vi "BRig_FPGA_v3,93.vi"() -> ()   [LabVIEW 2014]
uses:
  <vilib>/rvi/Emulation/niFpgaGetClockAttributes.vi
  <vilib>/rvi/Emulation/niFpgaSctlEmulationGetInTimedLoop.vi
  <vilib>/rvi/Emulation/niFpgaEmulationReportErrorSimple.vi
  <vilib>/rvi/eio/common/nirviEmuTemplateMethod_errors.vi
  <vilib>/rvi/Emulation/niFpgaCriticalErrorInLSC.vi
  <vilib>/eio/EIONode/EIONode.xnode
panel:
  out "fpga_solenoid_R":bool
  out "fpga_solenoid_L":bool
  out "fpga_laser2":bool
  out "fpga_laser1":bool
  in  "L2Led_ON":bool
  in  "L1Led_ON":bool
  in  "Rising(F)_or_Falling(T)":bool
  in  "Solenoid_trig_R":bool
  in  "Solenoid_trig_L":bool
  in  "Solenoid_nTotal_R":u32=100
  in  "Solenoid_nTotal_L":u32=100
  in  "L2Led_Baseline":bool
  in  "L1Led_Baseline":bool
  in  "CueLed_Baseline":bool
  in  "I_allReward":bool
  in  "AnaOut_1":u16
  in  "CueLed_Event":bool
  in  "CueLed_nValley":u32=100
  in  "CueLed_nPeak":u32=100
  in  "LC_Event_l2":bool
  in  "LC_Laser_l2":bool
  in  "LC_nShutter_l2":u32=100
  in  "LC_nValley_l2":u32=100
  in  "LC_nPeak_l2":u32=100
  in  "LR_wrong_nDelay_l2":u32
  in  "LR_reward_nDelay_l2":u32
  in  "LR_wrong_nTotal_l2":u32=100
  in  "LR_reward_nTotal_l2":u32=100
  in  "LR_wrong_laser_l2":bool
  in  "LR_wrong_Event_l2":bool
  in  "LR_reward_Laser_l2":bool
  in  "LR_reward_Event_l2":bool
  out "AnaIn_1":u16
  out "AnaIn_0":u16
  out "timeTrial_count":u32
  in  "timeTrial_trig":bool
  in  "k1__counter_per_ms":u16=100 min=100 max=40000 step=1
  in  "LC_nShutter_l1":u32=100
  in  "AnaOut_0":u16
  in  "LC_nValley_l1":u32=100
  in  "LC_nPeak_l1":u32=100
  in  "LC_Event_l1":bool
  in  "LR_wrong_nTotal_l1":u32=100
  in  "LR_wrong_nDelay_l1":u32
  in  "LR_reward_nTotal_l1":u32=100
  in  "LR_reward_nDelay_l1":u32
  in  "LR_reward_Event_l1":bool
  in  "LR_wrong_Event_l1":bool
  out "SelectWrong":bool
  out "SelectReward":bool
  in  "LR_wrong_Laser_l1":bool
  in  "LR_reward_Laser_l1":bool
  in  "Left(F)_or_Right(T)":bool
  in  "ignoreWrong":bool
  in  "SelectionState":bool
  in  "LC_Laser_l1":bool
  in  "FPGA_Stop":bool
  in  "audioTrigger_L":bool
  in  "audioTrigger_R":bool
  in  "audioFreq_L_kHz":u8=14 min=1 max=14 step=1
  in  "audioAmp_L":u16=1 min=1 max=32767 step=1
  in  "audioFreq_R_kHz":u8=14 min=1 max=14 step=1
  in  "audioAmp_R":u16=1 min=1 max=32767 step=1
  in  "A3_SL":bool
  in  "A1_SR":bool
  in  "Counts_Reset":bool
  out "A4_LickR":u32
  out "A2_LickL":u32
  in  "A6_Act":bool
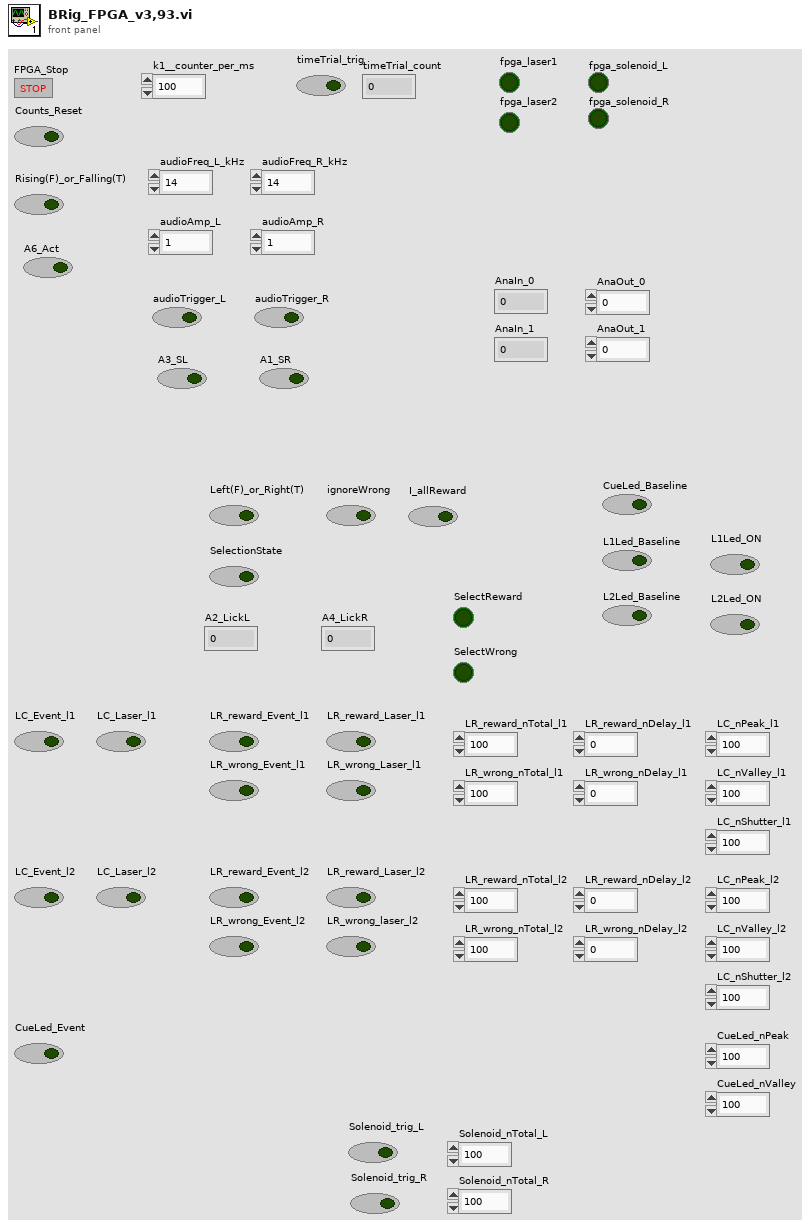
[diagram p1: front panel]
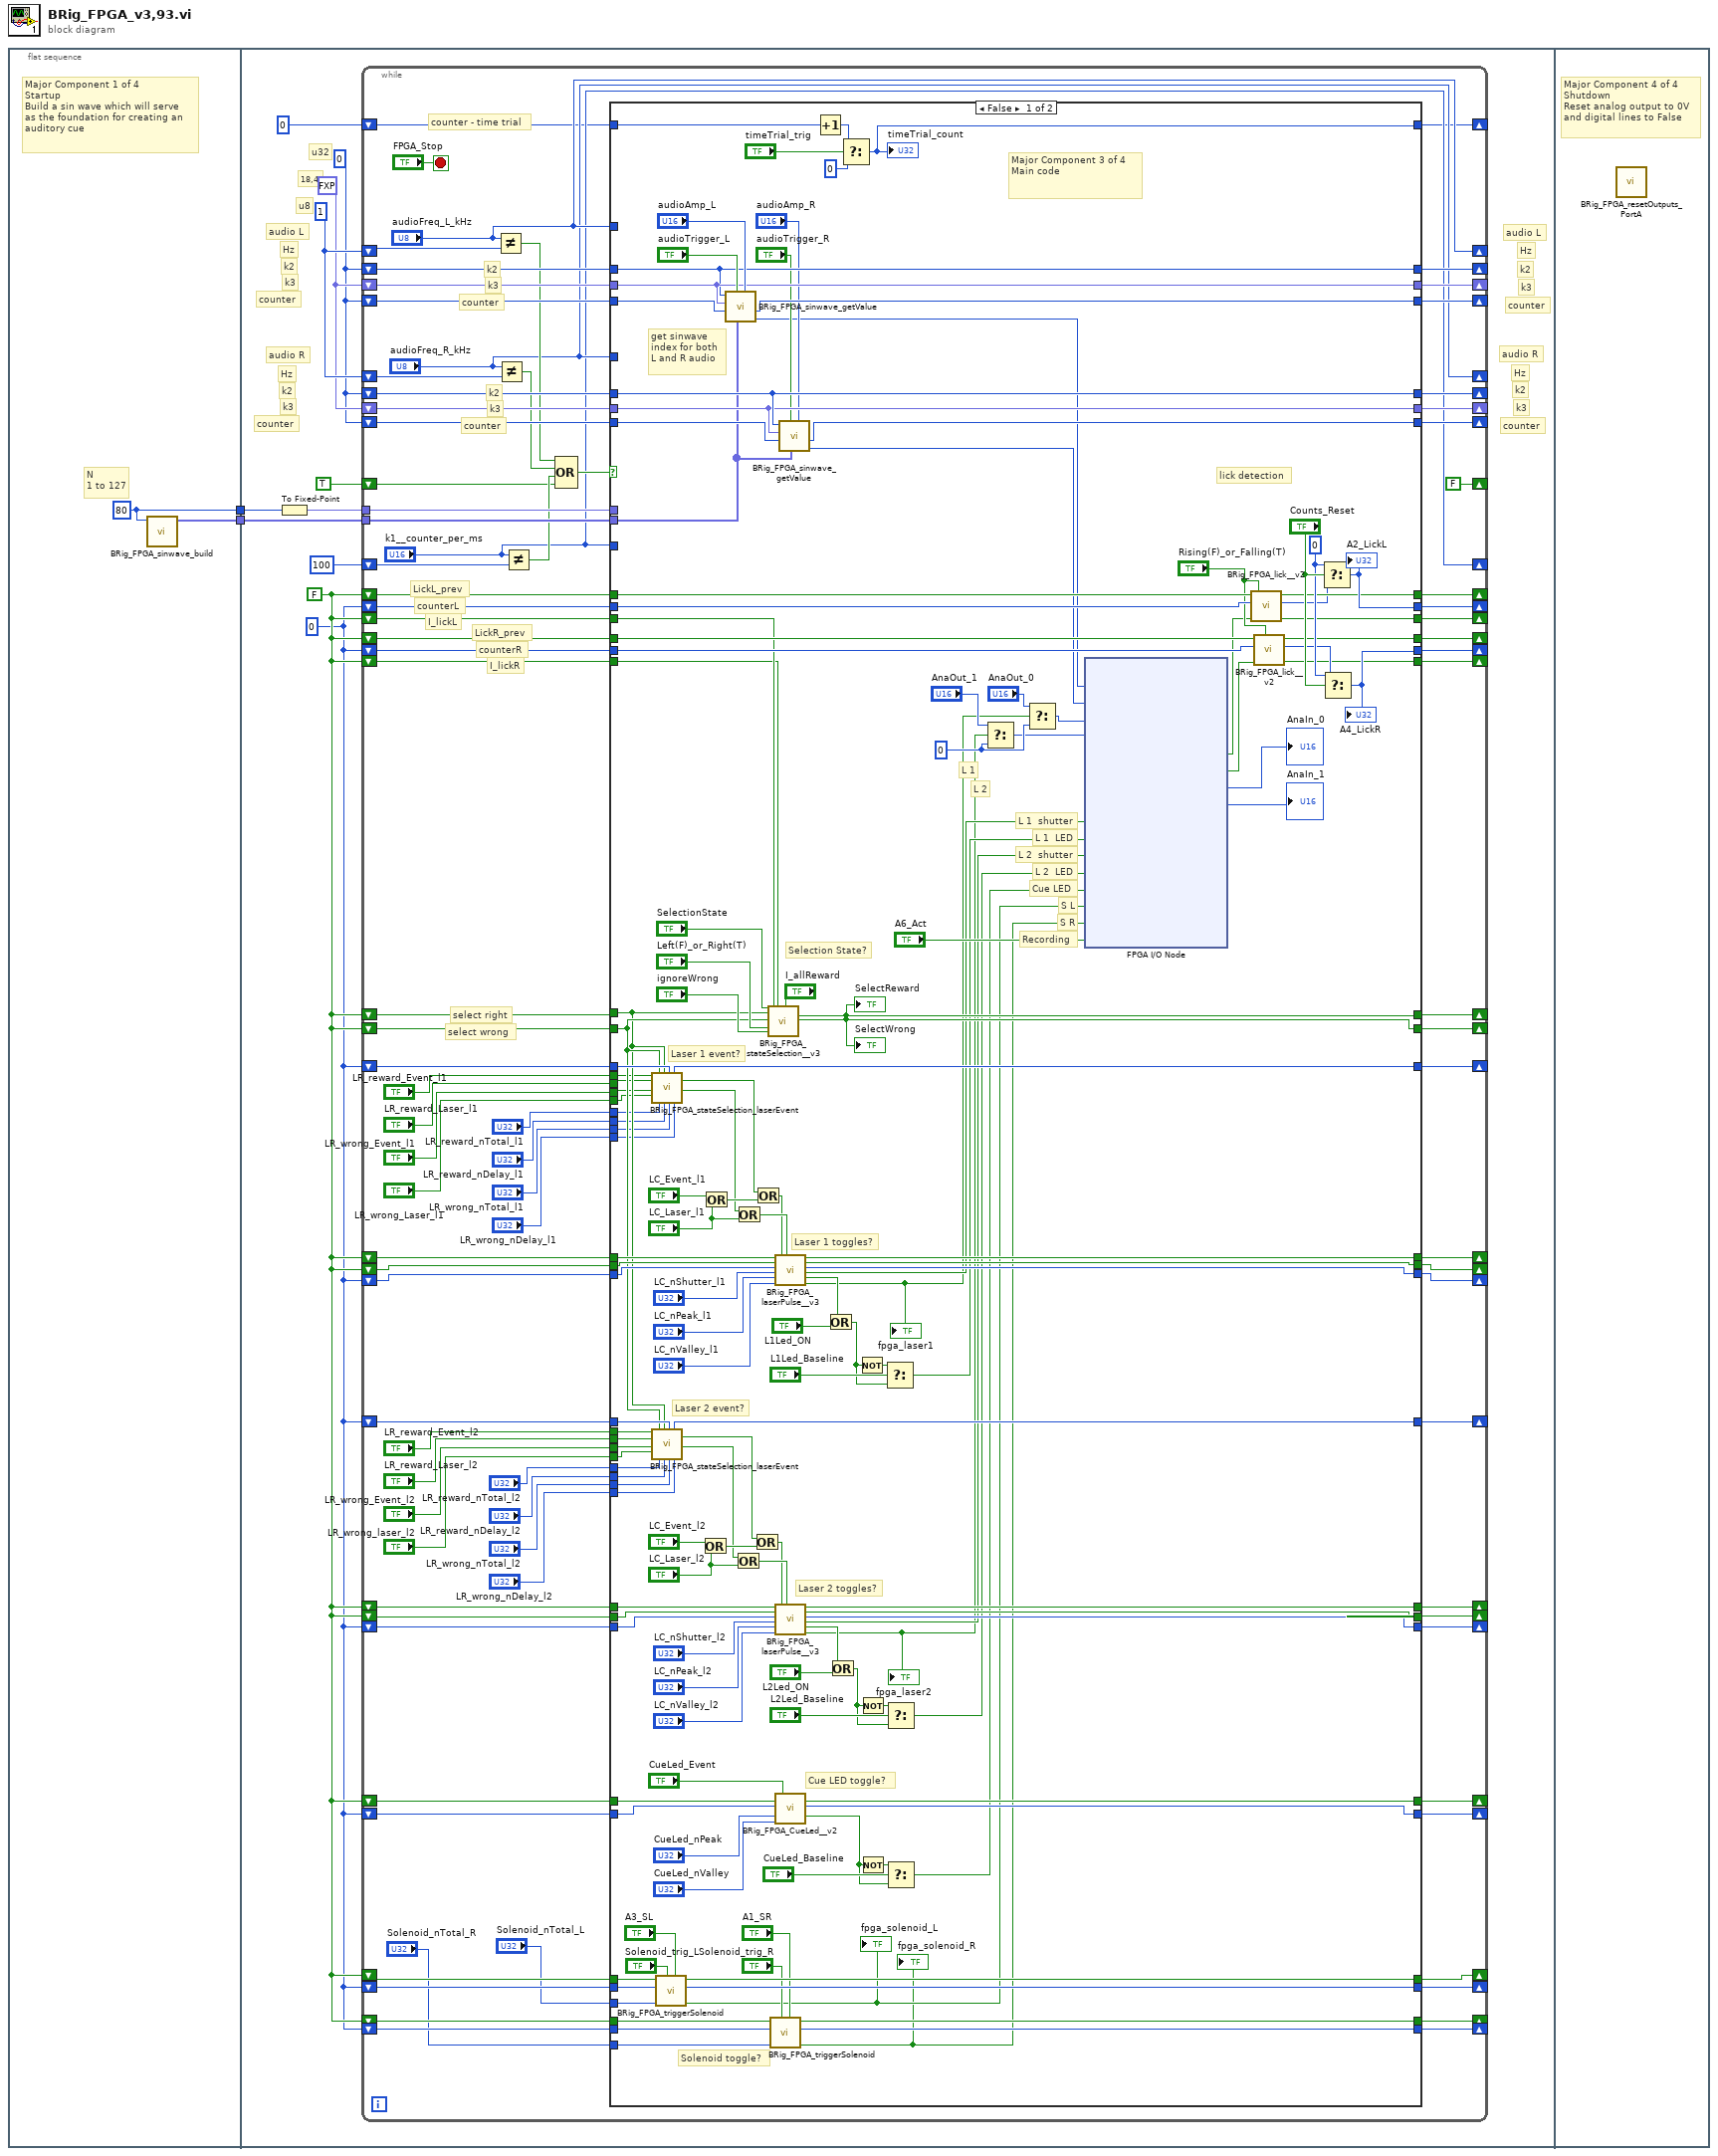
[diagram p0: block diagram]
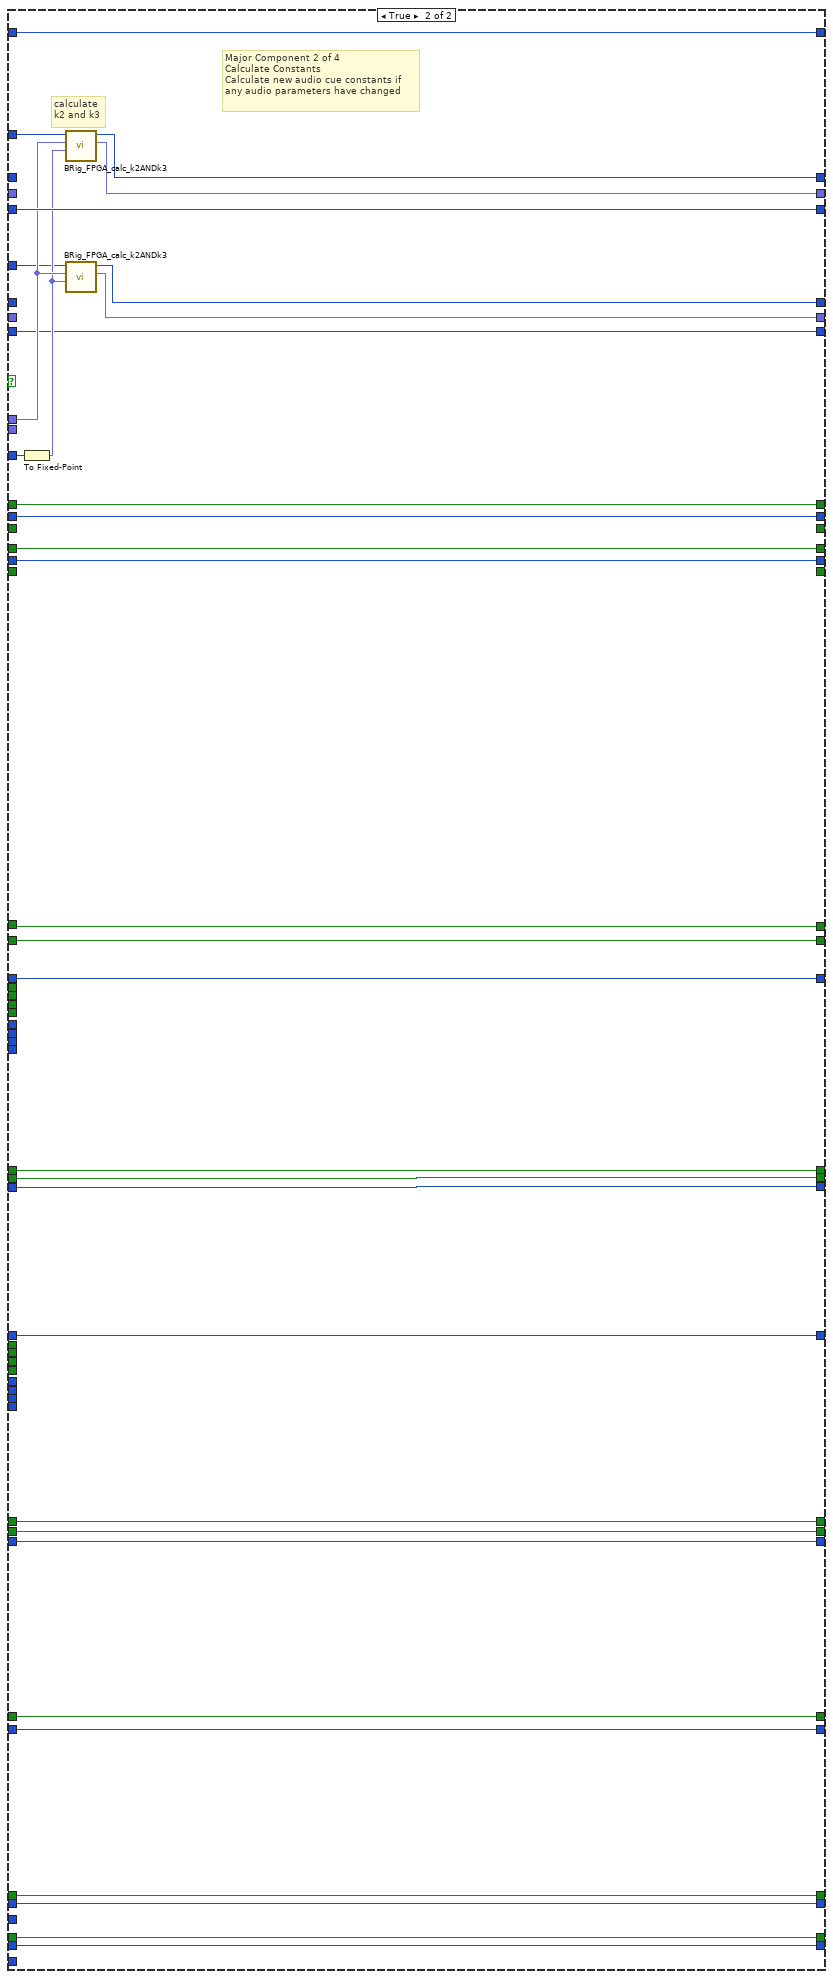
[diagram p2: hidden frame]
diagram:
  n1 = flat-sequence {
    tunnel: [w4] -> w2
    tunnel: [w3] -> w1
    tunnel: w2 -> [w15]
    tunnel: w1 -> [w14]
    frame #0 {
      w3 = 80 ("dimension size")
      # "Major Component 1 of 4\nStartup\nBuild a sin wave which will serve\nas the foundation for creating an\nauditory cue"
      # "N\n1 to 127"
      n2 = call "BRig_FPGA_sinwave_build.vi"("input_Npts"=w3) -> ("output_array_sin"=w4:fxp<+/-,16,2>[])  [unwired: 10 in]
    }
    frame #1 {
      w5 = u32 0
      w6 = FALSE
      w10 = u32 0
      w11 = fxp<+,18,4> 0.0
      w12 = u8 1
      # "counter"
      # "k3"
      # "k2"
      # "counter"
      # "k3"
      # "k2"
      # "counter"
      # "counter"
      # "u32"
      # "k3"
      # "k2"
      # "k3"
      # "18,4"
      # "u8"
      # "Hz"
      # "Hz"
      # "audio R"
      # "audio L"
      # "Hz"
      # "k2"
      # "Hz"
      # "audio R"
      # "audio L"
      n3 = To Fixed-Point(number=w14) -> (fixed-point=w13:fxp<+,7,7>)  [unwired: 1 in]
      n4 = while {
        shift-right: ["audioFreq_L_kHz"] -> _
        shift-left: w12 -> [w106]
        shift-right: [w100] -> _
        shift-left: w10 -> [w104]
        shift-right: ["audioFreq_R_kHz"] -> _
        shift-left: w12 -> [w96]
        tunnel: w15 -> [w103]
        tunnel: w13 -> [w102]
        shift-right: [w99] -> _
        shift-left: w11 -> [w101]
        shift-right: [w97] -> _
        shift-left: w10 -> [w98]
        shift-right: [w94] -> _
        shift-left: w10 -> [w95]
        shift-right: [w92] -> _
        shift-left: w11 -> [w93]
        shift-right: [w90] -> _
        shift-left: w10 -> [w91]
        shift-right: ["k1__counter_per_ms"] -> _
        shift-left: u16 100 ("y") -> [w89]
        shift-right: [FALSE] -> _
        shift-left: TRUE -> [w84]
        shift-right: [w77] -> _
        shift-left: w6 -> [w79]
        shift-right: [w76] -> _
        shift-left: w6 -> [w78]
        shift-right: [w74] -> _
        shift-left: w5 -> [w75]
        shift-right: [w72] -> _
        shift-left: w5 -> [w73]
        shift-right: [w69] -> _
        shift-left: w6 -> [w71]
        shift-right: [w68] -> _
        shift-left: w6 -> [w70]
        shift-right: [w66] -> _
        shift-left: w6 -> [w67]
        shift-right: [w64] -> _
        shift-left: w6 -> [w65]
        shift-right: [w62] -> _
        shift-left: u32 0 -> [w63]
        shift-right: [w60] -> _
        shift-left: w5 -> [w61]
        shift-right: [w59] -> _
        shift-left: w6 -> [w56]
        shift-right: [w58] -> _
        shift-left: w6 -> [w55]
        shift-right: [w57] -> _
        shift-left: w5 -> [w54]
        shift-right: [w52] -> _
        shift-left: w5 -> [w53]
        shift-right: [w51] -> _
        shift-left: w6 -> [w48]
        shift-right: [w50] -> _
        shift-left: w6 -> [w47]
        shift-right: [w49] -> _
        shift-left: w5 -> [w46]
        shift-right: [w45] -> _
        shift-left: w6 -> [w43]
        shift-right: [w44] -> _
        shift-left: w5 -> [w42]
        shift-right: [w24] -> _
        shift-left: w5 -> [w25]
        shift-right: [w21] -> _
        shift-left: w6 -> [w23]
        shift-right: [w18] -> _
        shift-left: w6 -> [w20]
        shift-right: [w17] -> _
        shift-left: w5 -> [w19]
        stop <- "FPGA_Stop" stop-if-true
        # "counter"
        # "k3"
        # "k2"
        # "counter"
        # "k3"
        # "k2"
        # "counter - time trial"
        # "I_lickR"
        # "counterR"
        # "LickR_prev"
        # "I_lickL"
        # "counterL"
        # "LickL_prev"
        # "select wrong"
        # "select right"
        n5 = Not Equal?(x="audioFreq_L_kHz", y=w106) -> (x != y?=w88:bool)
        n6 = Not Equal?(x="audioFreq_R_kHz", y=w96) -> (x != y?=w87:bool)
        n7 = Not Equal?(x="k1__counter_per_ms", y=w89) -> (x != y?=w85:bool)
        n8 = Compound Arithmetic op=OR(w88, w87, w85, w84) -> (w86:bool)
        n9 = case shown="False" w86 {
          tunnel: w104 -> [w241 _]
          tunnel: "audioFreq_L_kHz" -> [_ w287]
          tunnel: w103 -> [w234 _]
          tunnel: w102 -> [_ w283]
          tunnel: "k1__counter_per_ms" -> [_ w288]
          tunnel: w101 -> [w242 _]
          tunnel: [w241 w286] -> w100
          tunnel: [w242 w285] -> w99
          tunnel: w98 -> [w246 w284]
          tunnel: [w243 w284] -> w97
          tunnel: w95 -> [w238 _]
          tunnel: [w238 w279] -> w94
          tunnel: w93 -> [w237 _]
          tunnel: [w237 w280] -> w92
          tunnel: w91 -> [w240 w278]
          tunnel: "audioFreq_R_kHz" -> [_ w281]
          tunnel: [w239 w278] -> w90
          tunnel: w79 -> [w229 w277]
          tunnel: w78 -> [w228 w276]
          tunnel: [w233 w277] -> w77
          tunnel: [w226 w276] -> w76
          tunnel: w75 -> [w230 w275]
          tunnel: [w256 w275] -> w74
          tunnel: w73 -> [w227 w274]
          tunnel: [w253 w274] -> w72
          tunnel: w71 -> [w184 w273]
          tunnel: w70 -> [w185 w272]
          tunnel: [w204 w273] -> w69
          tunnel: [w249 w272] -> w68
          tunnel: [w219 w269] -> w59
          tunnel: [w220 w268] -> w58
          tunnel: [w221 w267] -> w57
          tunnel: w67 -> [w223 _]
          tunnel: [w232 _] -> w66
          tunnel: w65 -> [w222 _]
          tunnel: [w224 _] -> w64
          tunnel: w63 -> [w211 w271]
          tunnel: [w208 w271] -> w62
          tunnel: w61 -> [w203 w270]
          tunnel: [w202 w270] -> w60
          tunnel: w56 -> [w201 w269]
          tunnel: w55 -> [w200 w268]
          tunnel: w54 -> [w199 w267]
          tunnel: w53 -> [w187 w266]
          tunnel: [w186 w266] -> w52
          tunnel: [w182 w265] -> w51
          tunnel: [w181 w264] -> w50
          tunnel: [w180 w263] -> w49
          tunnel: w48 -> [w179 w265]
          tunnel: w47 -> [w178 w264]
          tunnel: w46 -> [w177 w263]
          tunnel: [w174 w262] -> w45
          tunnel: [w173 w261] -> w44
          tunnel: w43 -> [w172 w262]
          tunnel: w42 -> [w171 w261]
          tunnel: "LR_reward_Event_l1" -> [w157 _]
          tunnel: "LR_reward_Laser_l1" -> [w156 _]
          tunnel: "LR_wrong_Event_l1" -> [w155 _]
          tunnel: "LR_wrong_Laser_l1" -> [w154 _]
          tunnel: "LR_reward_nTotal_l1" -> [w153 _]
          tunnel: "LR_reward_nDelay_l1" -> [w152 _]
          tunnel: "LR_wrong_nTotal_l1" -> [w151 _]
          tunnel: "LR_wrong_nDelay_l1" -> [w150 _]
          tunnel: "LR_reward_Event_l2" -> [w149 _]
          tunnel: "LR_reward_Laser_l2" -> [w148 _]
          tunnel: "LR_wrong_Event_l2" -> [w147 _]
          tunnel: "LR_wrong_laser_l2" -> [w146 _]
          tunnel: "LR_reward_nTotal_l2" -> [w145 _]
          tunnel: "LR_reward_nDelay_l2" -> [w144 _]
          tunnel: "LR_wrong_nTotal_l2" -> [w143 _]
          tunnel: "LR_wrong_nDelay_l2" -> [w142 _]
          tunnel: w25 -> [w141 w260]
          tunnel: [w136 w260] -> w24
          tunnel: w23 -> [w140 w259]
          tunnel: "Solenoid_nTotal_L" -> [w139 _]
          tunnel: [w135 w259] -> w21
          tunnel: w20 -> [w132 w258]
          tunnel: w19 -> [w131 w257]
          tunnel: [w130 w258] -> w18
          tunnel: [w129 w257] -> w17
          tunnel: "Solenoid_nTotal_R" -> [w128 _]
          frame False {
            w168 = u16 0 ("f")
            w254 = u32 0 ("t")
            # "Cue LED"
            # "L 2  shutter"
            # "L 2  LED"
            # "L 1  shutter"
            # "L 1  LED"
            # "Recording"
            # "S L"
            # "S R"
            # "L 2"
            # "L 1"
            # "Solenoid toggle?"
            # "Cue LED toggle?"
            # "Laser 2 toggles?"
            # "Laser 2 event?"
            # "Laser 1 toggles?"
            # "Selection State?"
            # "Laser 1 event?"
            # "Major Component 3 of 4\nMain code"
            # "get sinwave\nindex for both\nL and R audio"
            # "lick detection"
            n10 = call "BRig_FPGA_stateSelection_laserEvent.vi"("I_LR_reward"=w157, "I_LR_reward_laser"=w156, "I_LR_wrong"=w155, "I_LR_wrong_laser"=w154, "I_selectWrong"=w185, "laser_reward_nTotal"=w153, "I_selectReward"=w184, "laser_reward_nDelay"=w152, "counter"=w203, "laser_wrong_nTotal"=w151, "laser_wrong_nDelay"=w150) -> ("output_counter"=w202:u32, "output_I_laserEvent"=w198:bool, "output_I_laserOn"=w197:bool)  [unwired: 6 in]
            n11 = call "BRig_FPGA_stateSelection_laserEvent.vi"("I_LR_reward"=w149, "I_LR_reward_laser"=w148, "I_LR_wrong"=w147, "I_LR_wrong_laser"=w146, "I_selectWrong"=w185, "laser_reward_nTotal"=w145, "I_selectReward"=w184, "laser_reward_nDelay"=w144, "counter"=w187, "laser_wrong_nTotal"=w143, "laser_wrong_nDelay"=w142) -> ("output_counter"=w186:u32, "output_I_laserEvent"=w183:bool, "output_I_laserOn"=w188:bool)  [unwired: 6 in]
            n12 = call "BRig_FPGA_triggerSolenoid.vi"("input_Solenoid_MTrig"="A3_SL", "input_Solenoid_trig"="Solenoid_trig_L", "input_threshold"=w139, "input_counter"=w141, "input_trig"=w140) -> ("output_Solenoid_OnOff"=w108:bool, "output_counter"=w136:u32, "output_trig"=w135:bool)  [unwired: 4 in]
            "fpga_solenoid_L" <- w108
            n13 = Or(x="LC_Event_l2", y="LC_Laser_l2") -> (x .or. y?=w192:bool)
            n14 = Or(x="LC_Event_l1", y="LC_Laser_l1") -> (x .or. y?=w215:bool)
            n15 = call "BRig_FPGA_sinwave_getValue.vi"("audioAmp"="audioAmp_L", "sinwave"=w234, "audioTrigger"="audioTrigger_L", "counter"=w246, "k3"=w242, "k2"=w241) -> ("output_audioValue"=w206:i16, "output_counter"=w243:u32)  [unwired: 4 in]
            n16 = Or(x=w188, y="LC_Laser_l2") -> (x .or. y?=w190:bool)
            n17 = Or(x=w197, y="LC_Laser_l1") -> (x .or. y?=w213:bool)
            n18 = Or(x=w183, y=w192) -> (x .or. y?=w189:bool)
            n19 = Or(x=w198, y=w215) -> (x .or. y?=w212:bool)
            n20 = call "BRig_FPGA_stateSelection__v3.vi"("I_selectionState"="SelectionState", "I_selectRight"=w184, "I_selectWrong"=w185, "I_Left(F)_or_Right(T)"="Left(F)_or_Right(T)", "I_ignoreWrong"="ignoreWrong", "I_lickL"=w223, "I_lickR"=w222, "I_allReward"="I_allReward") -> ("output__I_selectRight"=w204:bool, "output__I_selectWrong"=w249:bool)  [unwired: 18 in]
            "SelectWrong" <- w249
            "SelectReward" <- w204
            n21 = call "BRig_FPGA_triggerSolenoid.vi"("input_Solenoid_MTrig"="A1_SR", "input_Solenoid_trig"="Solenoid_trig_R", "input_threshold"=w128, "input_counter"=w131, "input_trig"=w132) -> ("output_Solenoid_OnOff"=w107:bool, "output_counter"=w129:u32, "output_trig"=w130:bool)  [unwired: 4 in]
            "fpga_solenoid_R" <- w107
            n22 = call "BRig_FPGA_laserPulse__v3.vi"("I_shutter"=w201, "I_peak"=w200, "count"=w199, "laser_Nshutter"="LC_nShutter_l1", "laser_Npeak"="LC_nPeak_l1", "laser_Nvalley"="LC_nValley_l1", "I_laserEvent"=w212, "I_laser"=w213) -> ("output_I_shutter"=w219:bool, "output_I_peak"=w220:bool, "output_count"=w221:u32, "output_shutter"=w115:bool, "output_led"=w125:bool, "output_laser"=w110:bool)  [unwired: 6 in]
            "fpga_laser1" <- w110
            n23 = call "BRig_FPGA_laserPulse__v3.vi"("I_shutter"=w179, "I_peak"=w178, "count"=w177, "laser_Nshutter"="LC_nShutter_l2", "laser_Npeak"="LC_nPeak_l2", "laser_Nvalley"="LC_nValley_l2", "I_laserEvent"=w189, "I_laser"=w190) -> ("output_I_shutter"=w182:bool, "output_I_peak"=w181:bool, "output_count"=w180:u32, "output_shutter"=w113:bool, "output_led"=w122:bool, "output_laser"=w109:bool)  [unwired: 6 in]
            "fpga_laser2" <- w109
            n24 = call "BRig_FPGA_CueLed__v2.vi"("I_peak"=w172, "count"=w171, "laser_Npeak"="CueLed_nPeak", "laser_Nvalley"="CueLed_nValley", "I_CueLed_Event"="CueLed_Event") -> ("output_I_peak"=w174:bool, "output_count"=w173:u32, "output_led"=w162:bool)  [unwired: 12 in]
            n25 = call "BRig_FPGA_sinwave_getValue.vi"("audioAmp"="audioAmp_R", "sinwave"=w234, "audioTrigger"="audioTrigger_R", "counter"=w240, "k3"=w237, "k2"=w238) -> ("output_audioValue"=w205:i16, "output_counter"=w239:u32)  [unwired: 4 in]
            n26 = Increment(x=w211) -> (x+1=w210:u32)
            n27 = Or(x=w125, y="L1Led_ON") -> (x .or. y?=w124:bool)
            n28 = Or(x=w122, y="L2Led_ON") -> (x .or. y?=w121:bool)
            n29 = Select(t=w210, s="timeTrial_trig", f=u32 0) -> (s? t:f=w208:u32)
            "timeTrial_count" <- w208
            n30 = Not(x=w124) -> (.not. x?=w161:bool)
            n31 = Not(x=w121) -> (.not. x?=w159:bool)
            n32 = Not(x=w162) -> (.not. x?=w164:bool)
            n33 = Select(t=w161, s="L1Led_Baseline", f=w124) -> (s? t:f=w114:bool)
            n34 = Select(t=w159, s="L2Led_Baseline", f=w121) -> (s? t:f=w112:bool)
            n35 = Select(t=w164, s="CueLed_Baseline", f=w162) -> (s? t:f=w111:bool)
            n36 = Select(t="AnaOut_1", s=w109, f=w168) -> (s? t:f=w166:u16)
            n37 = Select(t="AnaOut_0", s=w110, f=w168) -> (s? t:f=w169:u16)
            n38 = xnode "FPGA I/O Node"("AudioOut/Left"=w206, "AudioOut/Right"=w205, "ConnectorB/AO0"=w169, "ConnectorB/AO1"=w166, "ConnectorA/DIO6"=w115, "ConnectorB/DIO14"=w114, "ConnectorA/DIO7"=w113, "ConnectorB/DIO15"=w112, "ConnectorB/DIO9"=w111, "ConnectorA/DIO3"=w108, "ConnectorA/DIO5"=w107, "ConnectorA/DIO0"="A6_Act") -> ("ConnectorA/DIO4"=w120:bool, "ConnectorA/DIO2"=w119:bool, "ConnectorB/AI1"=→"AnaIn_0":u16, "ConnectorB/AI2"=→"AnaIn_1":u16)  [unwired: 16 in, 16 out]
            n39 = call "BRig_FPGA_lick__v2.vi"("Rising(F)_or_Falling(T)"="Rising(F)_or_Falling(T)", "I_stateDetector_new"=w120, "counter"=w230, "I_stateDetector_prev"=w229) -> ("output_I_lick"=w232:bool, "output_counter"=w231:u32, "output_I_stateDetector_prev"=w233:bool)  [unwired: 5 in]
            n40 = call "BRig_FPGA_lick__v2.vi"("Rising(F)_or_Falling(T)"="Rising(F)_or_Falling(T)", "I_stateDetector_new"=w119, "counter"=w227, "I_stateDetector_prev"=w228) -> ("output_I_lick"=w224:bool, "output_counter"=w225:u32, "output_I_stateDetector_prev"=w226:bool)  [unwired: 5 in]
            n41 = Select(t=w254, s="Counts_Reset", f=w231) -> (s? t:f=w256:u32)
            "A2_LickL" <- w256
            n42 = Select(t=w254, s="Counts_Reset", f=w225) -> (s? t:f=w253:u32)
            "A4_LickR" <- w253
          }
          frame True {
            # "Major Component 2 of 4\nCalculate Constants\nCalculate new audio cue constants if\nany audio parameters have changed"
            # "calculate\nk2 and k3"
            n43 = To Fixed-Point(number=w288) -> (fixed-point=w282:fxp<+,16,16>)  [unwired: 1 in]
            n44 = call "BRig_FPGA_calc_k2ANDk3.vi"("input_k1[count/ms]"=w282, "input_Npts"=w283, "input_freq[kHz]"=w287) -> ("output_k3"=w285:fxp<+,18,4>, "output_k2"=w286:u32)  [unwired: 7 in]
            n45 = call "BRig_FPGA_calc_k2ANDk3.vi"("input_k1[count/ms]"=w282, "input_Npts"=w283, "input_freq[kHz]"=w281) -> ("output_k3"=w280:fxp<+,18,4>, "output_k2"=w279:u32)  [unwired: 7 in]
          }
        }
      }
    }
    frame #2 {
      # "Major Component 4 of 4\nShutdown\nReset analog output to 0V\nand digital lines to False"
      n46 = call "BRig_FPGA_resetOutputs_PortA.vi"() -> ()  [unwired: 12 in]
    }
  }
